vi "TangoMove.vi"(7 "Direction":string, 8 "error in (no error)":errorcluster, 10 "TANGO":i32, 11 "StepWidth":dbl) -> (0 "error out":errorcluster, 3 "Position":dbl[](array[numeric]))   [LabVIEW 2018]
uses:
  <userlib>/Tango_DLL/Tango_DLL.lvlib
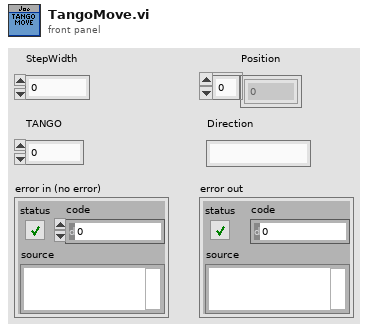
[diagram p1: front panel]
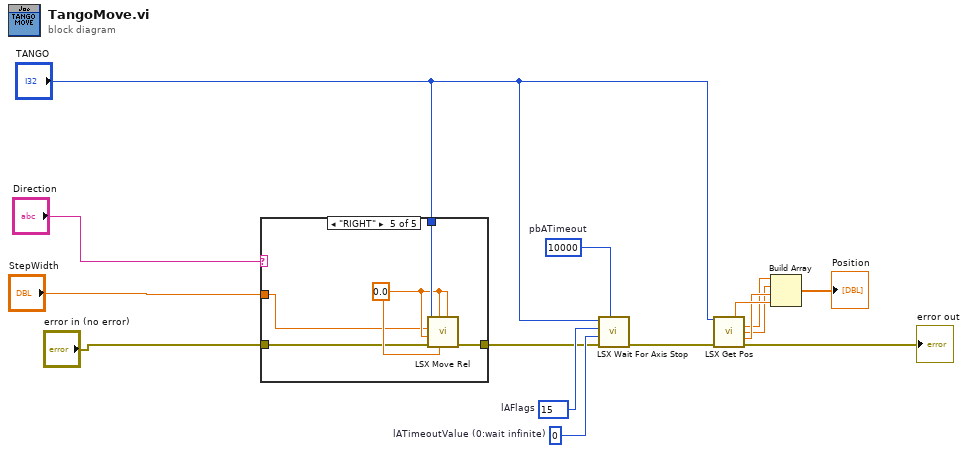
[diagram p0: block diagram]
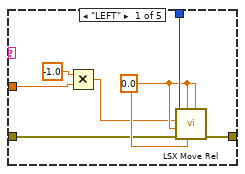
[diagram p2: hidden frame]
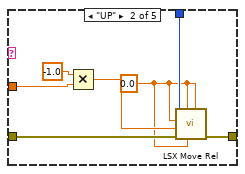
[diagram p3: hidden frame]
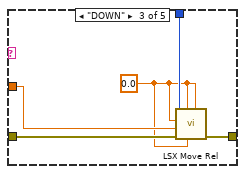
[diagram p4: hidden frame]
diagram:
  w15 = 10000  # pbATimeout
  w14 = i8 15  # lAFlags
  w13 = 0  # lATimeoutValue (0:wait infinite)
  n1 = case shown="\"RIGHT\"" "Direction" {
    tunnel: "TANGO" -> [w22 w29 w34 _ w40]
    tunnel: [w21 w28 w33 w35 w39] -> w10
    tunnel: "StepWidth" -> [w18 w27 w32 _ w37]
    tunnel: "error in (no error)" -> [w16 w25 w31 w35 w36]
    frame "LEFT" {
      w20 = 0.0 ("dY")
      n2 = Multiply(x=-1.0, y=w18) -> (x*y=w19:dbl)
      n3 = call <userlib>:"LSX Move Rel.vi"("bWait"=w20, "dA"=w20, "dZ"=w20, "error in (no error)"=w16, "dY"=w20, "dX"=w19, "lLSID"=w22) -> ("error out"=w21:errorcluster)  [unwired: 3 in, 1 out]
    }
    frame "UP" {
      w23 = 0.0 ("dY")
      n4 = Multiply(x=-1.0, y=w27) -> (x*y=w24:dbl)
      n5 = call <userlib>:"LSX Move Rel.vi"("bWait"=w23, "dA"=w23, "dZ"=w23, "error in (no error)"=w25, "dY"=w24, "dX"=w23, "lLSID"=w29) -> ("error out"=w28:errorcluster)  [unwired: 3 in, 1 out]
    }
    frame "DOWN" {
      w30 = 0.0 ("dY")
      n6 = call <userlib>:"LSX Move Rel.vi"("bWait"=w30, "dA"=w30, "dZ"=w30, "error in (no error)"=w31, "dY"=w32, "dX"=w30, "lLSID"=w34) -> ("error out"=w33:errorcluster)  [unwired: 3 in, 1 out]
    }
    frame "\u0000", Default {
    }
    frame "RIGHT" {
      w38 = 0.0 ("dY")
      n7 = call <userlib>:"LSX Move Rel.vi"("bWait"=w38, "dA"=w38, "dZ"=w38, "error in (no error)"=w36, "dY"=w38, "dX"=w37, "lLSID"=w40) -> ("error out"=w39:errorcluster)  [unwired: 3 in, 1 out]
    }
  }
  n8 = call <userlib>:"LSX Wait For Axis Stop.vi"("pbATimeout"=w15, "error in (no error)"=w10, "lATimeoutValue"=w13, "lAFlags"=w14, "lLSID"="TANGO") -> ("error out"=w12:errorcluster)  [unwired: 4 in, 2 out]
  n9 = call <userlib>:"LSX Get Pos.vi"("lLSID"="TANGO", "error in (no error)"=w12) -> ("pdA out"=w7:dbl, "pdX out"=w4:dbl, "pdY out"=w5:dbl, "pdZ out"=w6:dbl, "error out"=→"error out":errorcluster)  [unwired: 8 in, 1 out]
  n10 = Build Array(w4, w5, w6, w7) -> (→"Position":dbl[])
